vi "Template.vi"() -> ()   [LabVIEW 2020]
uses:
  _Template/_Template/_Template.lvclass
  _Shared/_Shared.lvlib
  _Shared/Tree/Tree.lvlib
panel:
  out "Target":string
  in  "Tree":string(tree)
  in  "OK":bool
  # "Disclaimer: Please consider committing changes before AND after this action."
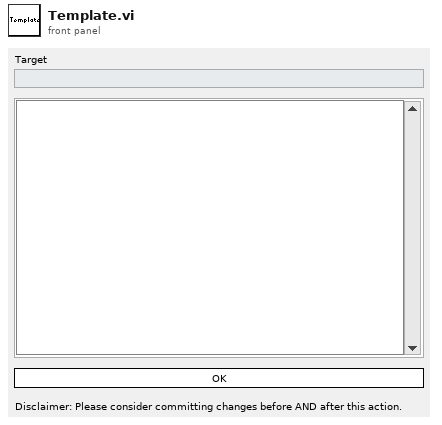
[diagram p1: front panel]
types:
  T1 = enum32{"Invalid", "Standard", "Closed", "Hidden", "Minimized", "Maximized"}
  T2 = typedef "_Shared.lvlib/Type Name Library File Path.ctl" = map{T3, T4}
  T3 = typedef "_Shared.lvlib/Type.ctl" = enum16{"Actor", "Msg"}
  T4 = typedef "_Shared.lvlib/Name Library File Path.ctl" = map{string, path}
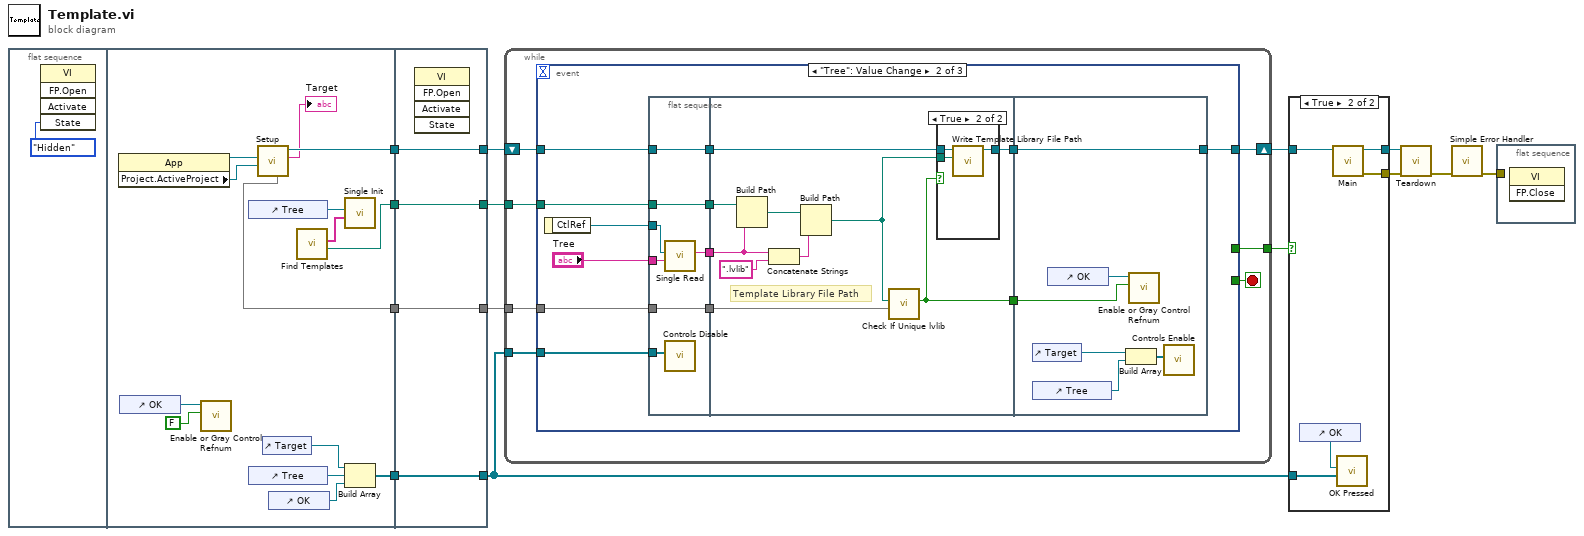
[diagram p0: block diagram]
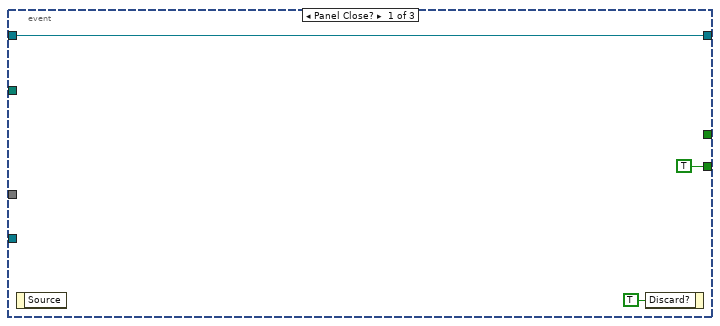
[diagram p2: hidden frame]
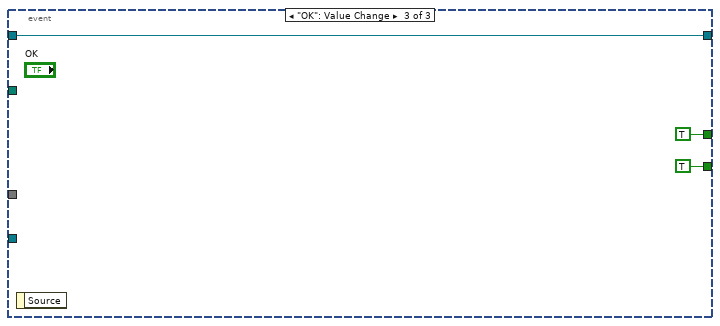
[diagram p4: hidden frame]
diagram:
  n1 = flat-sequence {
    tunnel: [w16] -> w12
    tunnel: [w28] -> w11
    tunnel: [w25] -> w7
    tunnel: [w20] -> w5
    tunnel: [w33] -> w9
    tunnel: w12 -> [w33]
    tunnel: [w32] -> w10
    tunnel: w11 -> [w32]
    tunnel: [w31] -> w8
    tunnel: w7 -> [w31]
    tunnel: [w30] -> w6
    tunnel: w5 -> [w30]
    frame #0 {
      n2 = invoke class="VI" method="FP.Open"("State"=T1."Hidden") -> ()  [unwired: 4 in, 5 out]
    }
    frame #1 {
      n3 = property class="App"() -> (reference out=w27:refnum<vi>, "Project.ActiveProject"=w26:refnum<vi>)  [unwired: 2 in, 1 out]
      n4 = control-ref of="OK"() -> (w23:refnum<vi>)
      n5 = call <vilib>:"Enable or Gray Control Refnum.vi"("enable?"=FALSE, "Control in"=w23) -> ()  [unwired: 8 in, 2 out]
      n6 = control-ref of="Tree"() -> (w21:refnum<vi>)
      n7 = control-ref of="Tree"() -> (w24:refnum<vi>)
      n8 = call "Setup.vi"("Active Project"=w26, "NI.LV.Dialog Instance"=w27) -> ("Target"=→"Target":string, "_Template out"=w25:refnum<class "_Template.lvclass">, "All Type Name Library File Path"=w16:T2)  [unwired: 6 in, 1 out]
      n9 = control-ref of="Target"() -> (w17:refnum<vi>)
      n10 = control-ref of="OK"() -> (w29:refnum<vi>)
      n11 = call "Find Templates.vi"() -> ("Template Path"=w20:path, "List Folders"=w19:string[])  [unwired: 10 in]
      n12 = call "Single Init.vi"("Left Cell Strings"=w19, "Tree Ref"=w21) -> ()  [unwired: 10 in]
      n13 = Build Array(w17, w24, w29) -> (w28:refnum<vi>[])
    }
    frame #2 {
      n14 = invoke class="VI" method="FP.Open"() -> ()  [unwired: 5 in, 5 out]
    }
  }
  n15 = while {
    tunnel: [w40] -> w14
    shift-right: [w37] -> w13
    shift-left: w8 -> [w38]
    tunnel: w6 -> [w36]
    tunnel: w9 -> [w35]
    tunnel: w10 -> [w34]
    stop <- w39 stop-if-true
    n16 = event shown="[1] \"Tree\": Value Change" {
      selector: _ -> [_ _ _]
      dyn-events: _ -> [_ _ _]
      timeout: _ -> [_ _ _]
      tunnel: [_ _ TRUE] -> w40
      tunnel: [TRUE ("Discard?") _ TRUE ("Discard?")] -> w39
      tunnel: w38 -> [w41 w50 w84]
      tunnel: [w41 w48 w84] -> w37
      tunnel: w36 -> [_ w52 _]
      tunnel: w35 -> [_ w54 _]
      tunnel: w34 -> [_ w56 _]
      event Panel Close? {
        n17 = event-data() -> ()  [unwired: 1 in, 1 out]
        n18 = event-data("Discard?"=TRUE) -> ()  [unwired: 1 in, 1 out]
      }
      event "Tree": Value Change {
        n19 = event-data() -> ("CtlRef"=w44:refnum<vi>)  [unwired: 1 in]
        n20 = flat-sequence {
          tunnel: w56 -> [w63]
          tunnel: [w62] -> w55
          tunnel: w54 -> [w62]
          tunnel: [w60] -> w53
          tunnel: w52 -> [w60]
          tunnel: [w61] -> w51
          tunnel: w50 -> [w61]
          tunnel: [w57] -> w49
          tunnel: "Tree" -> [w58]
          tunnel: w44 -> [w59]
          tunnel: w55 -> [w65]
          tunnel: w53 -> [w70]
          tunnel: w51 -> [w68]
          tunnel: w49 -> [w69]
          tunnel: [w67] -> w47
          tunnel: [w64] -> w46
          tunnel: [w83] -> w48
          tunnel: w47 -> [w83]
          tunnel: w46 -> [w81]
          frame #0 {
            n21 = call "Single Read.vi"("Tree"=w58, "Tree Ref"=w59) -> ("Cell String"=w57:string)  [unwired: 9 in]
            n22 = call "Controls Disable.vi"("Controls in"=w63) -> ()  [unwired: 11 in]
          }
          frame #1 {
            # "Template Library File Path"
            n23 = Build Path(base path=w70, name or relative path=w69) -> (appended path=w72:path)
            n24 = Concatenate Strings(w69, ".lvlib" ("string")) -> (w73:string)
            n25 = Build Path(base path=w72, name or relative path=w73) -> (appended path=w66:path)
            n26 = call "Check If Unique lvlib.vi"("All Type Name Library File Path"=w65, "Library File Path"=w66) -> ("Unique?"=w64:bool)  [unwired: 9 in]
            n27 = case shown="True" w64 {
              tunnel: w68 -> [w74 w77]
              tunnel: [w74 w76] -> w67
              tunnel: w66 -> [_ w75]
              frame False {
              }
              frame True {
                n28 = call "Write Template Library File Path.vi"("Template Library File Path"=w75, "_Template in"=w77) -> ("_Template out"=w76:refnum<class "_Template.lvclass">)  [unwired: 9 in]
              }
            }
          }
          frame #2 {
            n29 = control-ref of="Target"() -> (w80:refnum<vi>)
            n30 = control-ref of="Tree"() -> (w79:refnum<vi>)
            n31 = control-ref of="OK"() -> (w82:refnum<vi>)
            n32 = Build Array(w80, w79) -> (w78:refnum<vi>[])
            n33 = call <vilib>:"Enable or Gray Control Refnum.vi"("enable?"=w81, "Control in"=w82) -> ()  [unwired: 8 in, 2 out]
            n34 = call "Controls Enable.vi"("Controls in"=w78) -> ()  [unwired: 11 in]
          }
        }
      }
      event "OK": Value Change {
        n35 = event-data() -> ()  [unwired: 1 in, 1 out]
      }
    }
  }
  n36 = case shown="True" w14 {
    tunnel: w13 -> [w87 w89]
    tunnel: [_ w92] -> w4
    tunnel: w10 -> [_ w90]
    tunnel: [w87 w88] -> w2
    frame False {
    }
    frame True {
      n37 = control-ref of="OK"() -> (w91:refnum<vi>)
      n38 = call "Main.vi"("_Template in"=w89) -> ("error out"=w92:errorcluster, "_Template out"=w88:refnum<class "_Template.lvclass">)  [unwired: 9 in]
      n39 = call "OK Pressed.vi"("Controls in"=w90, "OK Ref"=w91) -> ()  [unwired: 10 in]
    }
  }
  n40 = call "Teardown.vi"("error in (no error)"=w4, "_Template in"=w2) -> ("error out"=w3:errorcluster)  [unwired: 9 in]
  n41 = call <vilib>:"Simple Error Handler.vi"("error in (no error)"=w3) -> ("error out"=w1:errorcluster)  [unwired: 4 in, 4 out]
  n42 = flat-sequence {
    tunnel: w1 -> [_]
    frame #0 {
      n43 = invoke class="VI" method="FP.Close"() -> ()  [unwired: 3 in, 3 out]
    }
  }
